vi "Number_recognition.vi"() -> ()   [LabVIEW 2013]
panel:
  in  "Reset":bool
  out "Weight":i64[][][](array[numeric])
  in  "Tab Control":enum32{"Learning", "Recognition"}(tab)
  out "Draw this number":i32
  in  "Pattern \nper number":i32
  out "Found":i32
  out "Result":i64[](array[numeric])
  in  "stop":bool
  out "Array":bool[][](array[boolean])
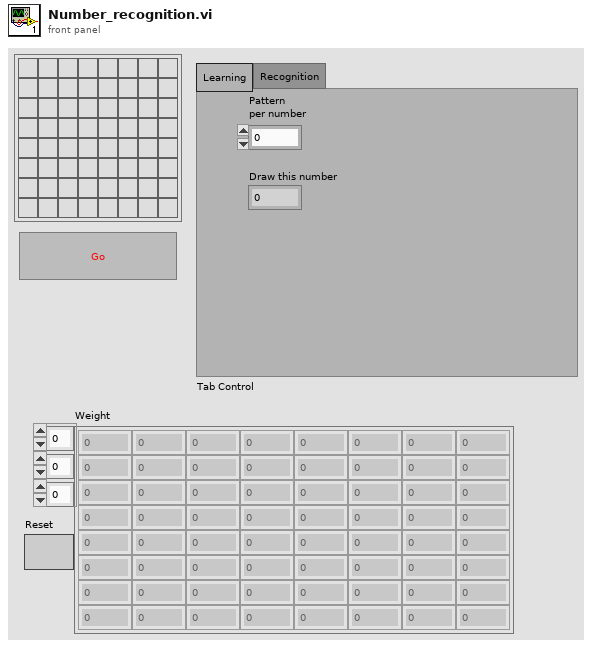
[diagram p1: front panel]
types:
  T1 = typedef "LVPoint32TypeDef.ctl" = cluster{"Horizontal":i32, "Vertical":i32}
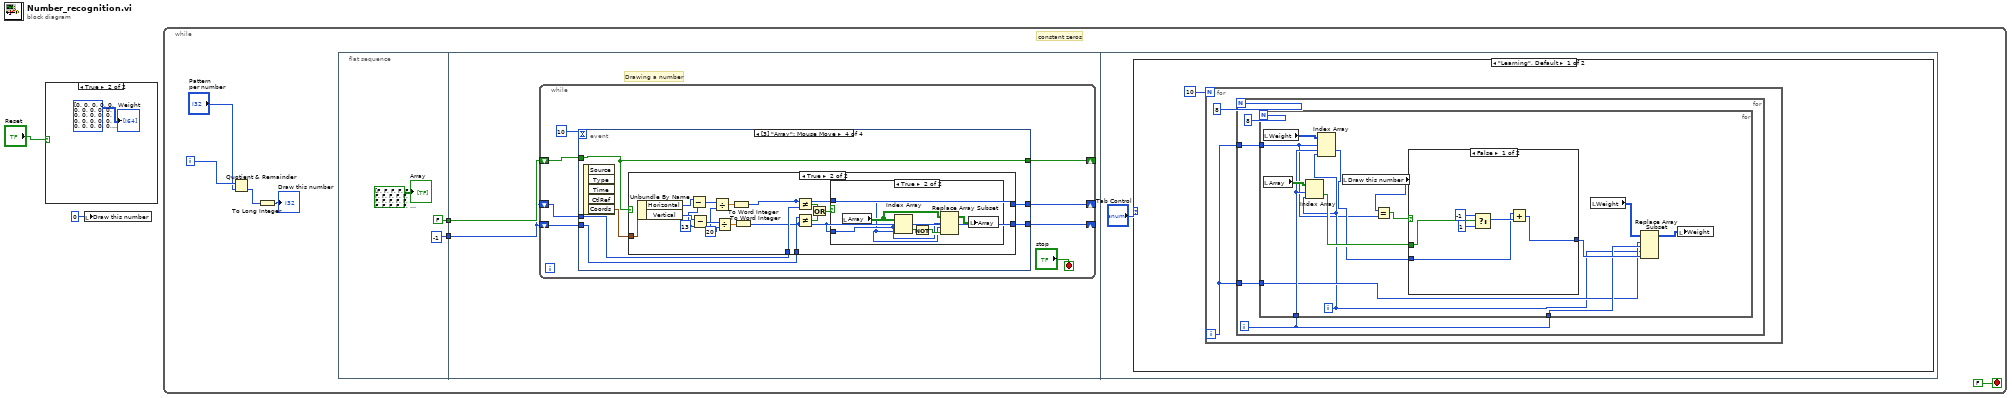
[diagram p0: block diagram]
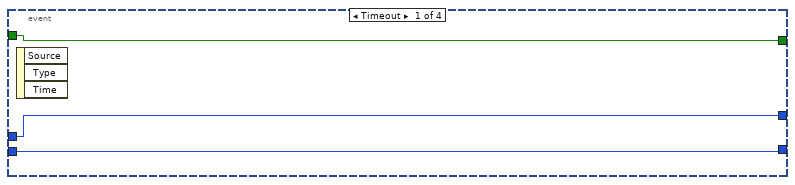
[diagram p3: hidden frame]
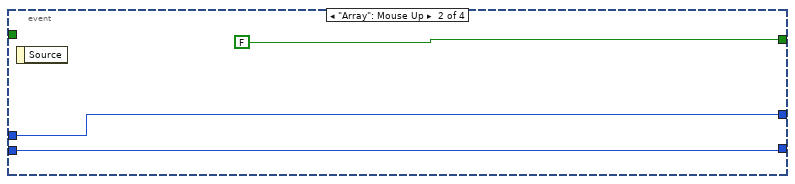
[diagram p4: hidden frame]
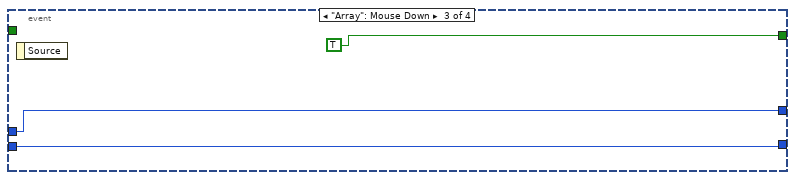
[diagram p5: hidden frame]
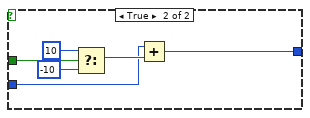
[diagram p8: hidden frame]
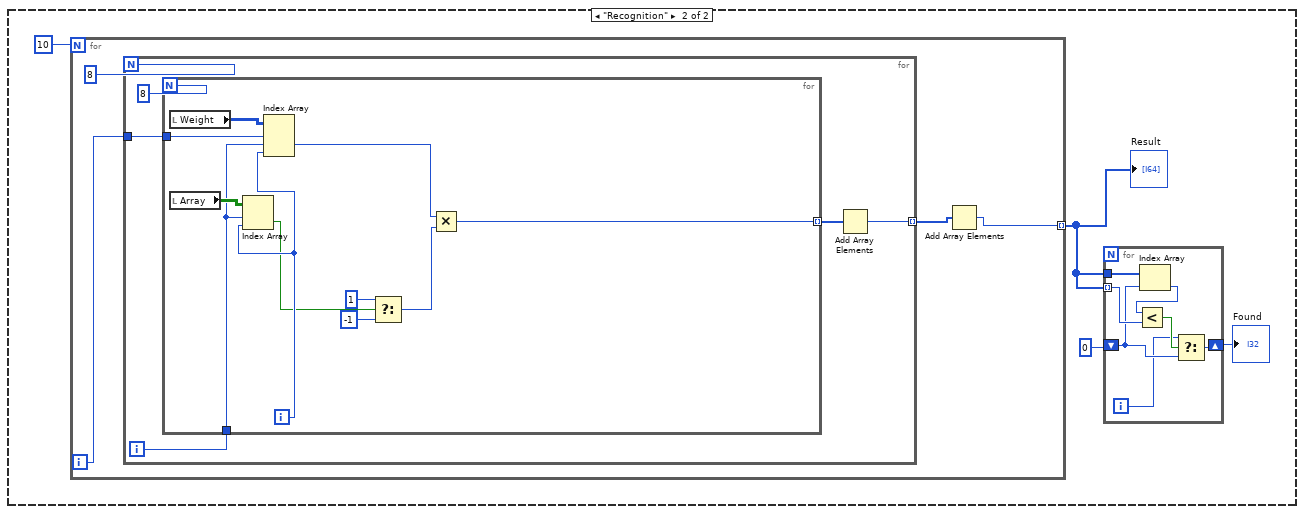
[diagram p9: hidden frame]
diagram:
  n1 = case shown="True" "Reset" {
    frame False {
    }
    frame True {
      "Weight" <- i32[][][] [[[0, 0, 0, 0, 0, 0, 0, 0], [0, 0, 0, 0, 0, 0, 0, 0], [0, 0, 0, 0, 0, 0, 0, 0], [0, 0, 0, 0, 0, 0, 0, 0], [0, 0, 0, 0, 0, 0, 0, 0], [0, 0, 0, 0, 0, 0, 0, 0], [0, 0, 0, 0, 0, 0, 0, 0], [0, 0, 0, 0, 0, 0, 0, 0]], [[0, 0, 0, 0, 0, 0, 0, 0], [0, 0, 0, 0, 0, 0, 0, 0], [0, 0, 0, 0, 0, 0, 0, 0], [0, 0, 0, 0, 0, 0, 0, 0], [0, 0, 0, 0, 0, 0, 0, 0], [0, 0, 0, 0, 0, 0, 0, 0], [0, 0, 0, 0, 0, 0, 0, 0], [0, 0, 0, 0, 0, 0, 0, 0]], [[0, 0, 0, 0, 0, 0, 0, 0], [0, 0, 0, 0, 0, 0, 0, 0], [0, 0, 0, 0, 0, 0, 0, 0], [0, 0, 0, 0, 0, 0, 0, 0], [0, 0, 0, 0, 0, 0, 0, 0], [0, 0, 0, 0, 0, 0, 0, 0], [0, 0, 0, 0, 0, 0, 0, 0], [0, 0, 0, 0, 0, 0, 0, 0]], [[0, 0, 0, 0, 0, 0, 0, 0], [0, 0, 0, 0, 0, 0, 0, 0], [0, 0, 0, 0, 0, 0, 0, 0], [0, 0, 0, 0, 0, 0, 0, 0], [0, 0, 0, 0, 0, 0, 0, 0], [0, 0, 0, 0, 0, 0, 0, 0], [0, 0, 0, 0, 0, 0, 0, 0], [0, 0, 0, 0, 0, 0, 0, 0]], [[0, 0, 0, 0, 0, 0, 0, 0], [0, 0, 0, 0, 0, 0, 0, 0], [0, 0, 0, 0, 0, 0, 0, 0], [0, 0, 0, 0, 0, 0, 0, 0], [0, 0, 0, 0, 0, 0, 0, 0], [0, 0, 0, 0, 0, 0, 0, 0], [0, 0, 0, 0, 0, 0, 0, 0], [0, 0, 0, 0, 0, 0, 0, 0]], [[0, 0, 0, 0, 0, 0, 0, 0], [0, 0, 0, 0, 0, 0, 0, 0], [0, 0, 0, 0, 0, 0, 0, 0], [0, 0, 0, 0, 0, 0, 0, 0], [0, 0, 0, 0, 0, 0, 0, 0], [0, 0, 0, 0, 0, 0, 0, 0], [0, 0, 0, 0, 0, 0, 0, 0], [0, 0, 0, 0, 0, 0, 0, 0]], [[0, 0, 0, 0, 0, 0, 0, 0], [0, 0, 0, 0, 0, 0, 0, 0], [0, 0, 0, 0, 0, 0, 0, 0], [0, 0, 0, 0, 0, 0, 0, 0], [0, 0, 0, 0, 0, 0, 0, 0], [0, 0, 0, 0, 0, 0, 0, 0], [0, 0, 0, 0, 0, 0, 0, 0], [0, 0, 0, 0, 0, 0, 0, 0]], [[0, 0, 0, 0, 0, 0, 0, 0], [0, 0, 0, 0, 0, 0, 0, 0], [0, 0, 0, 0, 0, 0, 0, 0], [0, 0, 0, 0, 0, 0, 0, 0], [0, 0, 0, 0, 0, 0, 0, 0], [0, 0, 0, 0, 0, 0, 0, 0], [0, 0, 0, 0, 0, 0, 0, 0], [0, 0, 0, 0, 0, 0, 0, 0]], [[0, 0, 0, 0, 0, 0, 0, 0], [0, 0, 0, 0, 0, 0, 0, 0], [0, 0, 0, 0, 0, 0, 0, 0], [0, 0, 0, 0, 0, 0, 0, 0], [0, 0, 0, 0, 0, 0, 0, 0], [0, 0, 0, 0, 0, 0, 0, 0], [0, 0, 0, 0, 0, 0, 0, 0], [0, 0, 0, 0, 0, 0, 0, 0]], [[0, 0, 0, 0, 0, 0, 0, 0], [0, 0, 0, 0, 0, 0, 0, 0], [0, 0, 0, 0, 0, 0, 0, 0], [0, 0, 0, 0, 0, 0, 0, 0], [0, 0, 0, 0, 0, 0, 0, 0], [0, 0, 0, 0, 0, 0, 0, 0], [0, 0, 0, 0, 0, 0, 0, 0], [0, 0, 0, 0, 0, 0, 0, 0]]] ("Weight")
    }
  }
  n2 = local write "Draw this number"(0 ("Draw this number")) -> ()
  n3 = while {
    i -> [w5]
    stop <- FALSE stop-if-true
    # "constant zeros"
    n4 = Quotient & Remainder(x=w5, y="Pattern \nper number") -> (floor(x/y)=w6:i32)  [unwired: 1 out]
    n5 = To Long Integer(number=w6) -> (32bit integer=→"Draw this number":i32)
    n6 = flat-sequence {
      tunnel: [FALSE] -> w10
      tunnel: [i16 -1] -> w9
      tunnel: w10 -> [w15]
      tunnel: w9 -> [w14]
      frame #0 {
        "Array" <- bool[][] [[FALSE, FALSE, FALSE, FALSE, FALSE, FALSE, FALSE, FALSE], [FALSE, FALSE, FALSE, FALSE, FALSE, FALSE, FALSE, FALSE], [FALSE, FALSE, FALSE, FALSE, FALSE, FALSE, FALSE, FALSE], [FALSE, FALSE, FALSE, FALSE, FALSE, FALSE, FALSE, FALSE], [FALSE, FALSE, FALSE, FALSE, FALSE, FALSE, FALSE, FALSE], [FALSE, FALSE, FALSE, FALSE, FALSE, FALSE, FALSE, FALSE], [FALSE, FALSE, FALSE, FALSE, FALSE, FALSE, FALSE, FALSE], [FALSE, FALSE, FALSE, FALSE, FALSE, FALSE, FALSE, FALSE]] ("Array")
      }
      frame #1 {
        # "Drawing a number"
        n7 = while {
          shift-right: [w21] -> _
          shift-left: w15 -> [w22]
          shift-right: [w18] -> _
          shift-left: w14 -> [w16]
          shift-right: [w19] -> _
          shift-left: w14 -> [w17]
          stop <- "stop" stop-if-true
          n8 = event shown="[3] \"Array\": Mouse Move" {
            selector: _ -> [_ _ _ _]
            dyn-events: _ -> [_ _ _ _]
            timeout: 10 -> [_ _ _ _]
            tunnel: w22 -> [w26 _ _ w38]
            tunnel: [w26 FALSE TRUE w38] -> w21
            tunnel: [w25 w28 w31 w36] -> w19
            tunnel: [w24 w27 w30 w35] -> w18
            tunnel: w17 -> [w25 w28 w31 w33]
            tunnel: w16 -> [w24 w27 w30 w34]
            event Timeout {
              n9 = event-data() -> ()  [unwired: 1 in, 3 out]
            }
            event "Array": Mouse Up {
              n10 = event-data() -> ()  [unwired: 1 in, 1 out]
            }
            event "Array": Mouse Down {
              n11 = event-data() -> ()  [unwired: 1 in, 1 out]
            }
            event "Array": Mouse Move {
              n12 = event-data() -> ("Coords"=w37:T1)  [unwired: 1 in, 4 out]
              n13 = case shown="True" w38 {
                tunnel: w37 -> [_ w56]
                tunnel: [w40 w42] -> w36
                tunnel: [w39 w41] -> w35
                tunnel: w34 -> [w39 w47]
                tunnel: w33 -> [w40 w46]
                frame False {
                }
                frame True {
                  w50 = 20
                  w53 = 13
                  n14 = Unbundle By Name(w56) -> ("Horizontal"=w55:i32, "Vertical"=w54:i32)
                  n15 = Subtract(x=w55, y=w53) -> (x-y=w52:i32)
                  n16 = Subtract(x=w54, y=w53) -> (x-y=w51:i32)
                  n17 = Divide(x=w52, y=w50) -> (x/y=w48:dbl)
                  n18 = Divide(x=w51, y=w50) -> (x/y=w49:dbl)
                  n19 = To Word Integer(number=w48) -> (16bit integer=w42:i16)
                  n20 = To Word Integer(number=w49) -> (16bit integer=w41:i16)
                  n21 = Not Equal?(x=w42, y=w46) -> (x != y?=w44:bool)
                  n22 = Not Equal?(x=w47, y=w41) -> (x != y?=w45:bool)
                  n23 = Or(x=w44, y=w45) -> (x .or. y?=w43:bool)
                  n24 = case shown="True" w43 {
                    tunnel: w42 -> [_ w57]
                    tunnel: w41 -> [_ w58]
                    frame False {
                    }
                    frame True {
                      n25 = local read "Array"() -> (w61:bool[][])
                      n26 = Index Array(array=w61, index (row)=w58, index (col)=w57) -> (element=w62:bool)
                      n27 = Not(x=w62) -> (.not. x?=w60:bool)
                      n28 = Replace Array Subset(array=w61, new element=w60, index (row)=w58, index (col)=w57) -> (w59:bool[][])
                      n29 = local write "Array"(w59) -> ()
                    }
                  }
                }
              }
            }
          }
        }
      }
      frame #2 {
        n30 = case shown="\"Learning\", Default" "Tab Control" {
          frame "Learning", Default {
            n31 = for {
              N: 10 -> [_]
              i -> [w65]
              n32 = for {
                N: 8 -> [_]
                tunnel: w65 -> [w70]
                tunnel: w65 -> [w68]
                i -> [w67]
                n33 = for {
                  N: 8 -> [_]
                  tunnel: w70 -> [w74]
                  tunnel: w67 -> [w81]
                  tunnel: w68 -> [w72]
                  tunnel: w67 -> [w77]
                  i -> [w73]
                  n34 = local read "Weight"() -> (w79:i64[][][])
                  n35 = local read "Array"() -> (w78:bool[][])
                  n36 = Index Array(array=w78, index (row)=w77, index (col)=w73) -> (element=w76:bool)
                  n37 = Index Array(array=w79, index (dim 0)=w72, index (dim 1)=w77, index (dim 2)=w73) -> (element=w75:i64)
                  n38 = local read "Draw this number"() -> (w71:i32)
                  n39 = Equal?(x=w71, y=w72) -> (x = y?=w84:bool)
                  n40 = case shown="False" w84 {
                    tunnel: w76 -> [w87 w96]
                    tunnel: w75 -> [w86 w92]
                    tunnel: [w85 w91] -> w82
                    frame False {
                      n41 = Select(t=-1, s=w87, f=1) -> (s? t:f=w88:i32)
                      n42 = Add(x=w86, y=w88) -> (x+y=w85:i64)
                    }
                    frame True {
                      n43 = Select(t=10, s=w96, f=-10) -> (s? t:f=w93:i32)
                      n44 = Add(x=w92, y=w93) -> (x+y=w91:i64)
                    }
                  }
                  n45 = local read "Weight"() -> (w83:i64[][][])
                  n46 = Replace Array Subset(array=w83, new element=w82, index (dim 0)=w74, index (dim 1)=w81, index (dim 2)=w73) -> (w80:i64[][][])
                  n47 = local write "Weight"(w80) -> ()
                }
              }
            }
          }
          frame "Recognition" {
            n48 = for {
              N: 10 -> [_]
              tunnel: [w108] -> w98 mode=indexing
              i -> [w110]
              n49 = for {
                N: 8 -> [_]
                tunnel: w110 -> [w115]
                tunnel: [w112] -> w109 mode=indexing
                i -> [w114]
                n50 = for {
                  N: 8 -> [_]
                  tunnel: w115 -> [w123]
                  tunnel: w114 -> [w125]
                  tunnel: [w117] -> w113 mode=indexing
                  i -> [w124]
                  n51 = local read "Weight"() -> (w127:i64[][][])
                  n52 = local read "Array"() -> (w126:bool[][])
                  n53 = Index Array(array=w126, index (row)=w125, index (col)=w124) -> (element=w122:bool)
                  n54 = Index Array(array=w127, index (dim 0)=w123, index (dim 1)=w125, index (dim 2)=w124) -> (element=w118:i64)
                  n55 = Select(t=1, s=w122, f=-1) -> (s? t:f=w119:i32)
                  n56 = Multiply(x=w118, y=w119) -> (x*y=w117:i64)
                }
                n57 = Add Array Elements(numeric array=w113) -> (sum=w112:i64)
              }
              n58 = Add Array Elements(numeric array=w109) -> (sum=w108:i64)
            }
            "Result" <- w98
            n59 = for {
              tunnel: w98 -> [w104] mode=indexing
              shift-right: [w107] -> w97
              shift-left: 0 -> [w102]
              tunnel: w98 -> [w106]
              i -> [w101]
              n60 = Index Array(array=w106, index=w102) -> (element=w105:i64)
              n61 = Less?(x=w105, y=w104) -> (x < y?=w103:bool)
              n62 = Select(t=w101, s=w103, f=w102) -> (s? t:f=w107:i32)
            }
            "Found" <- w97
          }
        }
      }
    }
  }
